vi "GLIMPSE get default acquisition file names.vi"(6 "error in":errorcluster, 9 "RAID root path":path=path "c:/scratch") -> (0 "error out":errorcluster, 1 "all directory names":string[](array[string]), 2 "next directory path":path, 3 "last directory path":path)   [LabVIEW 2016]
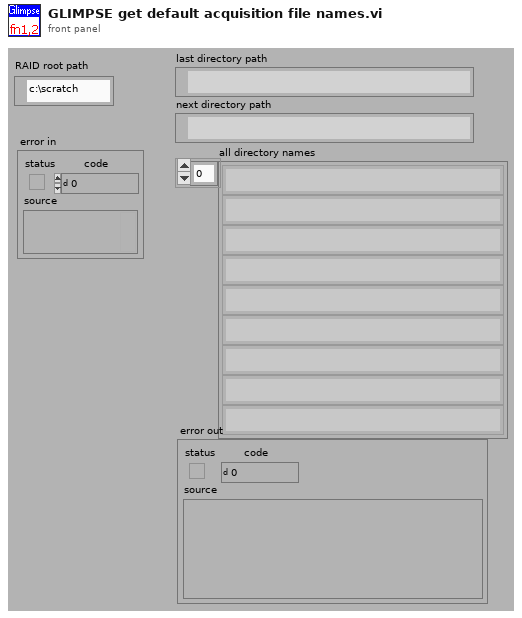
[diagram p1: front panel]
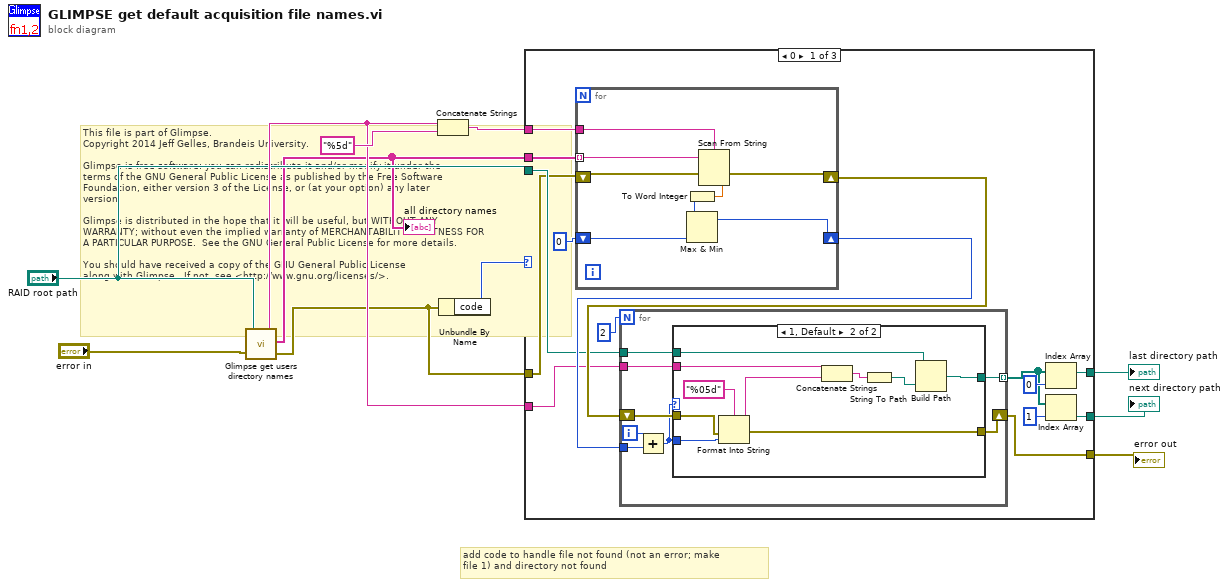
[diagram p0: block diagram]
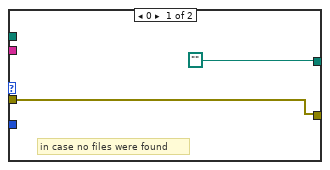
[diagram p2: hidden frame]
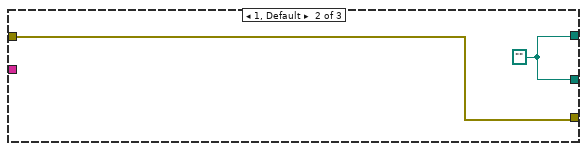
[diagram p3: hidden frame]
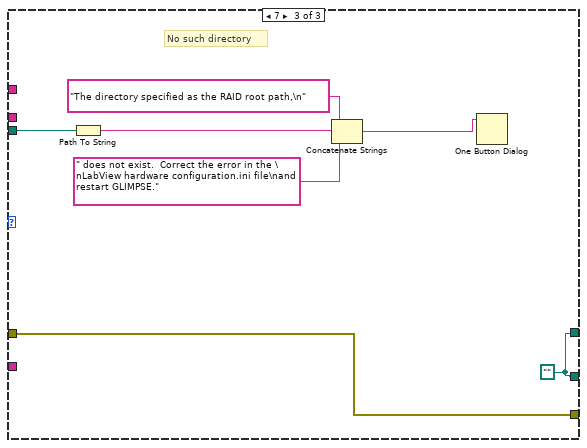
[diagram p4: hidden frame]
diagram:
  # "This file is part of Glimpse. \nCopyright 2014 Jeff Gelles, Brandeis University.    \n\nGlimpse is free software: you can redistribute it and/or modify it under the \nterms of the GNU General Public License as published by the Free Software \nFoundation, either version 3 of the License, or (at your option) any later \nversion.\n\nGlimpse is distributed in the hope that it will be useful, but WITHOUT ANY \nWARRANTY; without even the implied warranty of MERCHANTABILITY or FITNESS FOR \nA PARTICULAR PURPOSE.  See the GNU General Public License for more details.\n\nYou should have received a copy of the GNU General Public License\nalong with Glimpse.  If not, see <http://www.gnu.org/licenses/>."
  # "add code to handle file not found (not an error; make \nfile 1) and directory not found"
  n1 = call "Glimpse get users directory names.vi"("RAID root path"="RAID root path", "error in"="error in") -> ("Username"=w7:string, "directory names"=w1:string[], "error out"=w5:errorcluster)
  "all directory names" <- w1
  n2 = Concatenate Strings(w7, "%5d" ("string")) -> (w9:string)
  n3 = Unbundle By Name(w5) -> ("code"=w8:i32)
  n4 = case shown="0" w8 {
    tunnel: w1 -> [w26 _ _]
    tunnel: w9 -> [w25 _ _]
    tunnel: w7 -> [w20 _ _]
    tunnel: [w16 w56 w63] -> w6
    tunnel: w5 -> [w12 w56 w63]
    tunnel: "RAID root path" -> [w13 _ w58]
    tunnel: [w15 w55 w57] -> w3
    tunnel: [w14 w55 w57] -> w2
    frame 0 {
      n5 = for {
        tunnel: w26 -> [w54] mode=indexing
        tunnel: w25 -> [w53]
        shift-right: [w51] -> w21
        shift-left: w12 -> [w52]
        shift-right: [w48] -> w22
        shift-left: i16 0 -> [w49]
        n6 = Scan From String(format string=w53, input string=w54, error in=w52) -> (error out=w51:errorcluster, output 1=w50:dbl)  [unwired: 1 in, 3 out]
        n7 = To Word Integer(number=w50) -> (16bit integer=w47:i16)
        n8 = Max & Min(x=w47, y=w49) -> (max(x,y)=w48:i16)  [unwired: 1 out]
      }
      n9 = for {
        N: 2 -> [_]
        tunnel: w22 -> [w34]
        shift-right: [w31] -> w16
        shift-left: w21 -> [w32]
        tunnel: w20 -> [w30]
        tunnel: [w29] -> w17 mode=indexing
        tunnel: w13 -> [w27]
        i -> [w33]
        n10 = Add(x=w33, y=w34) -> (x+y=w28:i32)
        n11 = case shown="1, Default" w28 {
          tunnel: w28 -> [_ w46]
          tunnel: w32 -> [w35 w44]
          tunnel: [w35 w43] -> w31
          tunnel: w30 -> [_ w42]
          tunnel: [path "" w38] -> w29
          tunnel: w27 -> [_ w37]
          frame 0 {
            # "in case no files were found"
          }
          frame 1, Default {
            n12 = Format Into String(format string="%05d", error in=w44, w46) -> (resulting string=w41:string, error out=w43:errorcluster)  [unwired: 1 in]
            n13 = Concatenate Strings(w42, w41) -> (w40:string)
            n14 = String To Path(string=w40) -> (path=w39:path)
            n15 = Build Path(base path=w37, name or relative path=w39) -> (appended path=w38:path)
          }
        }
      }
      n16 = Index Array(array=w17, index=0) -> (element=w15:path)
      n17 = Index Array(array=w17, index=1) -> (element=w14:path)
    }
    frame 1, Default {
      w55 = path ""
    }
    frame 7 {
      w57 = path ""
      # "No such directory"
      n18 = Path To String(path=w58) -> (string=w62:string)
      n19 = Concatenate Strings("The directory specified as the RAID root path,\n", w62, " does not exist.  Correct the error in the \nLabView hardware configuration.ini file\nand restart GLIMPSE.") -> (w59:string)
      n20 = One Button Dialog(message=w59) -> ()  [unwired: 2 out]
    }
  }
  "error out" <- w6
  "next directory path" <- w2
  "last directory path" <- w3
